vi "Calibration correction.vi"(3 "new zero field coeff":T1(array[cluster])=[{"note"="7th_6T", "start"=1.8739770702937149, "end"=2.8092971732964953, "Tn coeffs"=[2.3040095380306127, -0.8959412253732818, 0.02084020508860851, 0.02995665860931248, -0.0017793974641133429, -0.00474186684486187, 0.0008132503860309566]}, {"note"="7th_6T", "start"=0.30101870386065765, "end"=2.0413970280813296, "Tn coeffs"=[4.662162773058288, -0.4524556325299596, 0.009701818190255855, -0.016288562353399576, 0.0011149333686050992, 0.0009558364086849862, 0.00021314049130340327]}], 5 "old T":dbl=20000.0 format="%.2f", 7 "old zero field coef":T1(array[cluster])=[{"note"="7th_6T", "start"=1.8739770702937149, "end"=2.8092971732964953, "Tn coeffs"=[2.3040095380306127, -0.8959412253732818, 0.02084020508860851, 0.02995665860931248, -0.0017793974641133429, -0.00474186684486187, 0.0008132503860309566]}, {"note"="7th_6T", "start"=0.30101870386065765, "end"=2.0413970280813296, "Tn coeffs"=[4.662162773058288, -0.4524556325299596, 0.009701818190255855, -0.016288562353399576, 0.0011149333686050992, 0.0009558364086849862, 0.00021314049130340327]}]) -> (1 "new T":dbl=0.2918892703761924)   [LabVIEW 2025]
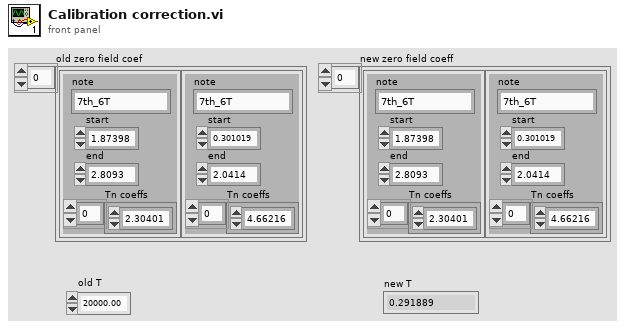
[diagram p1: front panel]
types:
  T1 = cluster{"note":string, "start":dbl, "end":dbl, "Tn coeffs":dbl[]}[]
  T2 = cluster{"note":string, "start":dbl, "end":dbl, "Tn coeffs":dbl[]}
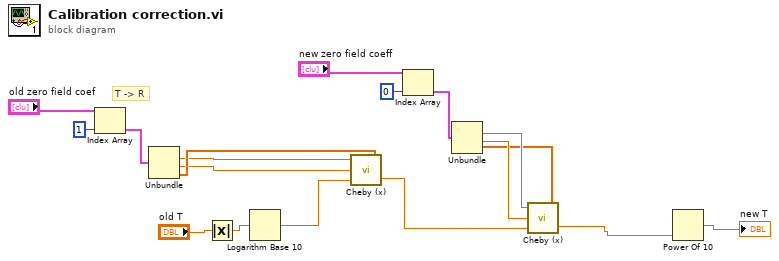
[diagram p0: block diagram]
diagram:
  # "T -> R"
  n1 = Index Array(array="old zero field coef", index=1) -> (element=w11:T2)
  n2 = Unbundle(w11) -> ("start"=w13:dbl, "end"=w12:dbl, "Tn coeffs"=w14:dbl[])  [unwired: 1 out]
  n3 = Absolute Value(x="old T") -> (abs(x)=w16:dbl)
  n4 = Logarithm Base 10(1:w16) -> (0:w15:dbl)
  n5 = call "Cheby (x).vi"("Tn coeffs"=w14, "x"=w15, "end"=w12, "start"=w13) -> ("f(x)"=w10:dbl)
  n6 = Index Array(array="new zero field coeff", index=0) -> (element=w8:T2)
  n7 = Unbundle(w8) -> ("start"=w6:dbl, "end"=w5:dbl, "Tn coeffs"=w4:dbl[])  [unwired: 1 out]
  n8 = call "Cheby (x).vi"("Tn coeffs"=w4, "x"=w10, "end"=w5, "start"=w6) -> ("f(x)"=w3:dbl)
  n9 = Power Of 10(x=w3) -> (10^x=→"new T":dbl)
